vi "Achizitie date.vi"() -> ()   [LabVIEW 2019]
uses:
  <vilib>/MakerHub/LINX/Public/Peripherals/Analog/Analog Read 1 Chan.vi
  <vilib>/MakerHub/LINX/Public/Peripherals/Analog/Analog Read N Chans.vi
  <vilib>/MakerHub/LINX/Private/Local IO/LinxAnalogRead.vi
  <vilib>/MakerHub/LINX/Public/Utilities/Check Channel.vi
  <vilib>/MakerHub/LINX/Public/Utilities/Open Serial.vi
  <vilib>/MakerHub/LINX/Private/Utilties/Generate Error.vi
  <vilib>/MakerHub/LINX/LMH-LINX.lvlib
panel:
  out "Semnalul 3":dbl(graph)
  out "Semnalul 2":dbl(graph)
  out "Semnalul 1":dbl(graph)
  out "Semnalul 4":dbl(graph)
  out "Voltage 4":dbl
  out "AI Ref 4":dbl
  out "AI Ref 3":dbl
  out "Voltage 3":dbl
  out "Voltage 2":dbl
  out "AI Ref 2":dbl
  out "Numeric":i32
  out "Voltage":dbl
  out "AI Ref":dbl
  in  "stop":bool
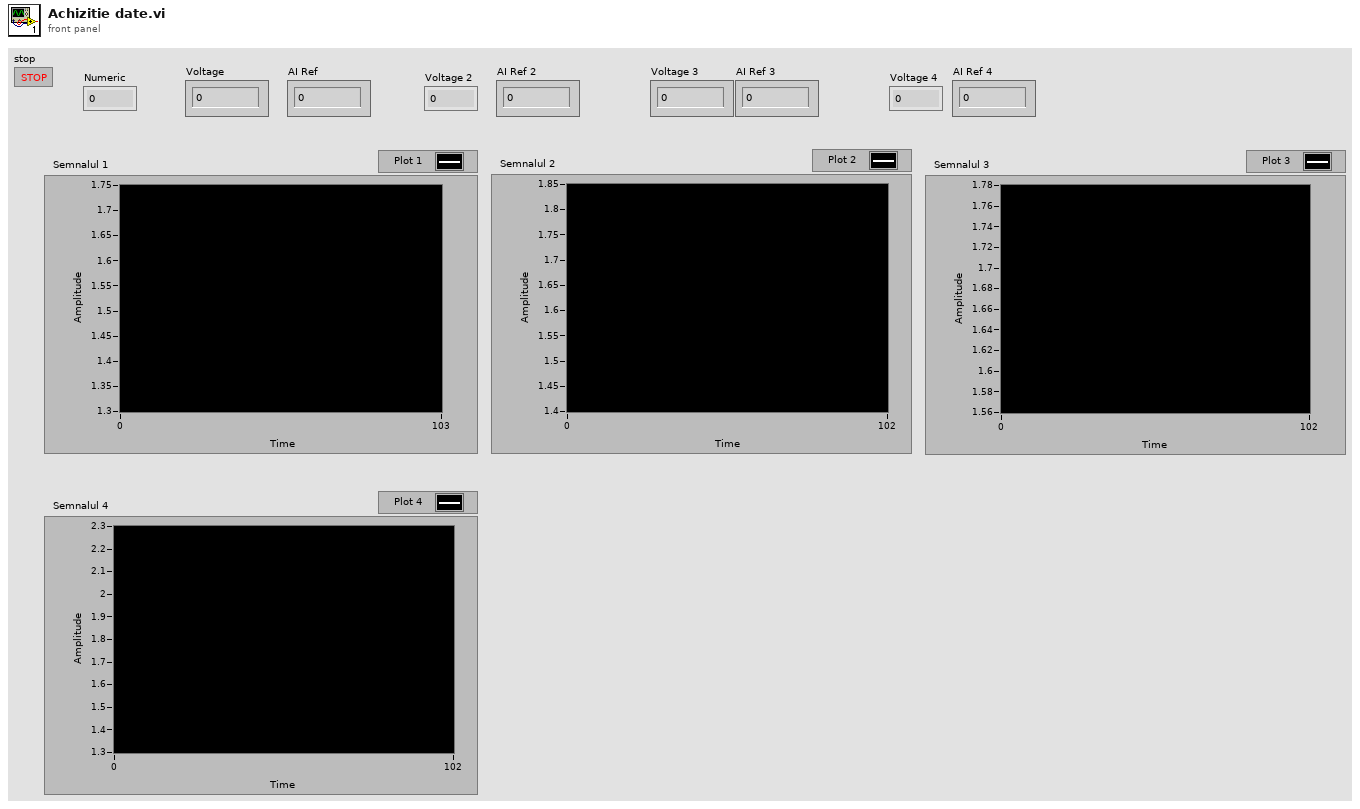
[diagram p1: front panel]
types:
  T1 = typedef "LMH-LINX.lvlib/LINX Ref.ctl" = cluster{"IO":T2, "Interface":T3, "LINX Device Config":T4}
  T2 = typedef "LMH-LINX.lvlib/Platform.ctl" = enum16{"Remote", "Local"}
  T3 = typedef "LMH-LINX.lvlib/Interface.ctl" = enum16{"Serial", "TCP"}
  T4 = typedef "LMH-LINX.lvlib/Device.lvlib/LINX Device Config.ctl" = cluster{"Interface":T3, "COM Port":refnum<visa-resource-name>, "TCP Configuration":T5, "Device Family":u8, "Device ID":u8, "Device Name":string, "TCP Ref":refnum<k5>, "Channels":T6}
  T5 = typedef "LMH-LINX.lvlib/Device.lvlib/TCP Config.ctl" = cluster{"IP Address":string, "Port":u16}
  T6 = typedef "LMH-LINX.lvlib/Channels.ctl" = cluster{"DI":u8[], "DO":u8[], "AI":u8[], "AO":u8[], "PWM":u8[], "QE":u8[], "UART":u8[], "I2C 2":u8[], "SPI":u8[], "CAN":u8[], "Servo":u8[], "AI Ref (V)":dbl, "AI Resolution (Bits)":u8, "AO Ref (V)":dbl, "AO Resolution (Bits)":u8}
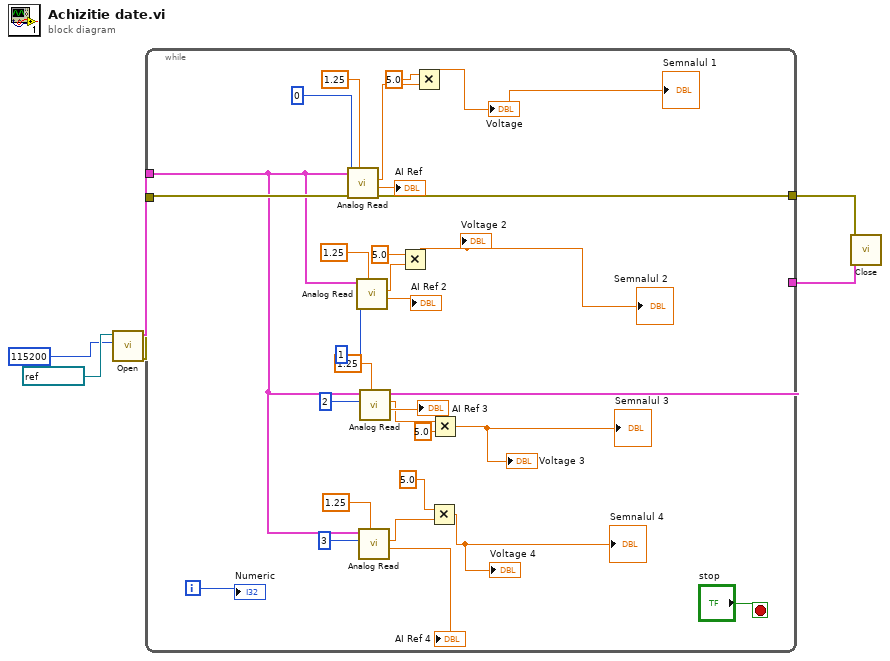
[diagram p0: block diagram]
diagram:
  n1 = call-poly <vilib>:"Open.vi"("Baud Rate Override"=u32 115200, "Serial Port"=refnum<visa-resource-name> "COM6") -> ("Error Out"=w3:errorcluster, "LINX Resource"=w4:T1)  [unwired: 7 in, 1 out]
  n2 = while {
    tunnel: w4 -> [w17]
    tunnel: w3 -> [w34]
    tunnel: [w11] -> w2
    tunnel: [w23] -> w1
    i -> [w33]
    stop <- "stop" stop-if-true
    n3 = call-poly <vilib>:"Analog Read.vi"("Analog Ref Override (V)"=1.25, "Error In"=w34, "Analog Channel"=u8 0, "LINX Resource"=w17) -> ("Error Out"=w11:errorcluster, "AI Ref"=→"AI Ref":dbl, "Voltage"=w29:dbl)  [unwired: 4 in, 1 out]
    n4 = call-poly <vilib>:"Analog Read.vi"("Analog Ref Override (V)"=1.25, "Analog Channel"=u8 1, "LINX Resource"=w17) -> ("AI Ref"=→"AI Ref 2":dbl, "Voltage"=w26:dbl)  [unwired: 5 in, 2 out]
    n5 = call-poly <vilib>:"Analog Read.vi"("Analog Ref Override (V)"=1.25, "Analog Channel"=u8 3, "LINX Resource"=w17) -> ("AI Ref"=→"AI Ref 4":dbl, "Voltage"=w13:dbl)  [unwired: 5 in, 2 out]
    n6 = call-poly <vilib>:"Analog Read.vi"("Analog Ref Override (V)"=1.25, "Analog Channel"=u8 2, "LINX Resource"=w17) -> ("AI Ref"=→"AI Ref 3":dbl, "Voltage"=w19:dbl, "LINX Resource"=w23:T1)  [unwired: 5 in, 1 out]
    n7 = Multiply(x=5.0, y=w26) -> (x*y=→"Voltage 2" →"Semnalul 2":dbl)
    n8 = Multiply(x=5.0, y=w29) -> (x*y=→"Voltage" →"Semnalul 1":dbl)
    n9 = Multiply(x=5.0, y=w13) -> (x*y=→"Voltage 4" →"Semnalul 4":dbl)
    n10 = Multiply(x=w19, y=5.0) -> (x*y=→"Voltage 3" →"Semnalul 3":dbl)
    "Numeric" <- w33
  }
  n11 = call <vilib>:"Close.vi"("Error In"=w2, "LINX Resource"=w1) -> ()  [unwired: 9 in, 1 out]
